vi "NI-DAQmxMulti.vi"() -> (0 "error out":errorcluster)   [LabVIEW 2022 SP3]
uses:
  Device ID port info.ctl
  Sub_vis/Upload Data.ctl
  <vilib>/DAQmx/read.llb/DAQmx Read (Analog 2D DBL NChan NSamp).vi
  Globals/Meas_global.vi
  <vilib>/DAQmx/miscellaneous.llb/DAQmx Fill In Error Info.vi
  <resource>/objmgr/daqmx.rc
panel:
  out "errorLog":T1(array[cluster])
  out "FsArray":dbl[](array[numeric]) format="%_12g"
  out "combinedTasks":string[](array[string])
  out "Device port info":T2[](array[typedef])
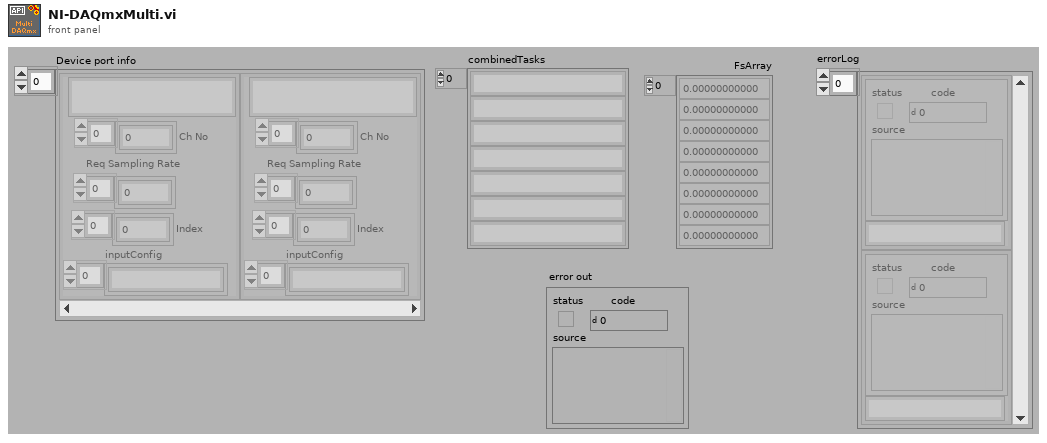
[diagram p1: front panel]
types:
  T1 = cluster{"error out":errorcluster, "String":string}[]
  T2 = typedef "Device ID port info.ctl" = cluster{"Ch No":i16[], "Req Sampling Rate":dbl[], "Port":string, "Index":i32[], "inputConfig":string[]}
  T3 = typedef "Analysis_info_cluster.ctl" = cluster{"Colour":u32, "Inst type":T4, "Inst name":string, "Symbol":string, "Code name":string, "Extra Info":string, "Inst Array":T5, "U":dbl, "u^2":dbl, "u^3":dbl, "u^4":dbl, "Skew_u":dbl, "Kurt_u":dbl, "Sd Error in Mean":dbl, "% u'/U":dbl, "X":dbl, "Y":dbl, "Z":dbl, "Timescale integral Estimate":dbl, "Sd Error in Variance":dbl, "Calib File":path, "Calib Constants":dbl[], "Output Position":bool, "Stats":enum16{"None", "Basic", "Full"}, "Av Sampling Rate":dbl, "Av No of Samples":dbl, "Total Meas Time (s)":dbl, "OrigChName":string, "Max value":dbl, "Min value":dbl, "Req Sample Rate Hz":dbl, "Sync Delay Time (s)":dbl, "Ch No":i16, "Device":string, "Use Latest Calib":bool, "Port":string, "Metadata Ch Names":string[], "Metadata Ch Values":string[], "Label":string, "chState":T6, "Point Drift":dbl, "inputConfig":string}
  T4 = typedef "Inst_type.ctl" = enum16{"Raw voltage", "Raw with zero offsetting", "Propeller anemometer", "Pressure Transducer", "Pitot-static tube", "Hot wire", "Cross wire 1", "Cross wire 2", "Generic Linear", "Generic Polynomial", "Generic BackPoly", "Fast FID", "Thermocouple", "Cold wire", "Pulsed Wire", "LDA Vel", "LDA Tran time", "LDA Arr time", "Microphone"}
  T5 = typedef "Instrument_Array.ctl" = enum16{"PWA", "LDA", "Analogue"}
  T6 = typedef "channelState.ctl" = enum32{"No Selection", "Solo", "Mute"}
  T7 = typedef "Upload Data.ctl" = enum16{"Voltage Array", "Time Trace Cluster"}
  T8 = typedef "Rendezvous RefNum" = refnum<k1>
  T9 = typedef "Setup.ctl" = enum16{"Run Program", "Show Setup", "Save Current Setup", "Setup Front Panel"}
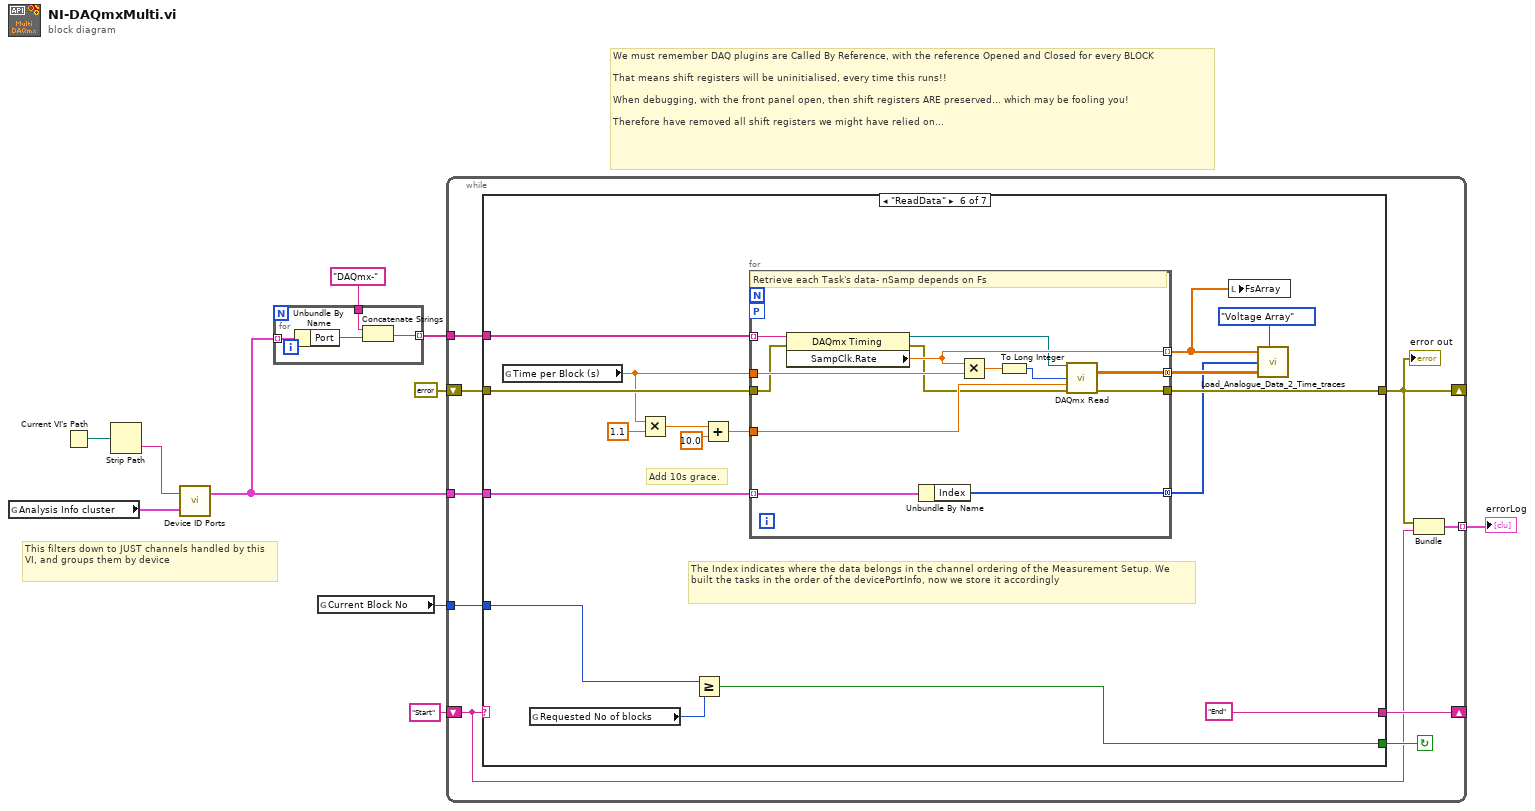
[diagram p0: block diagram]
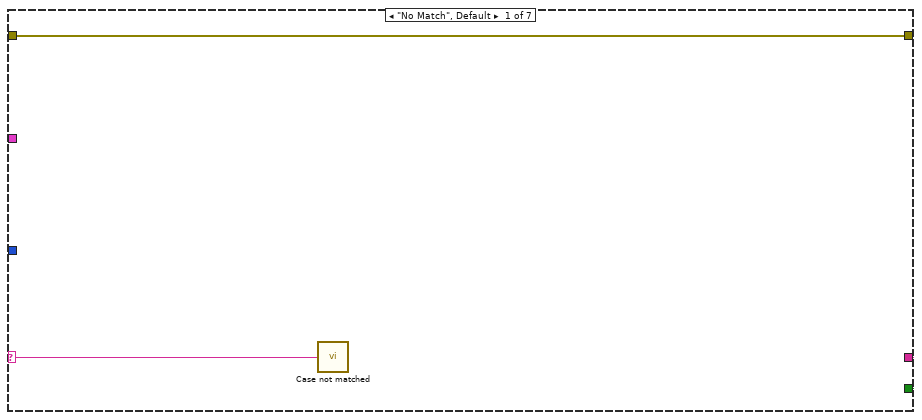
[diagram p2: hidden frame]
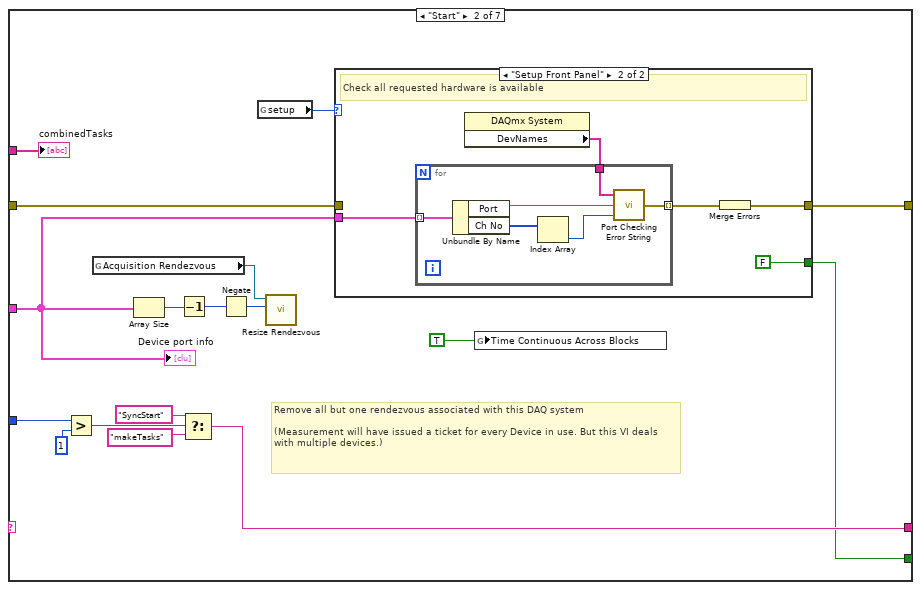
[diagram p3: hidden frame]
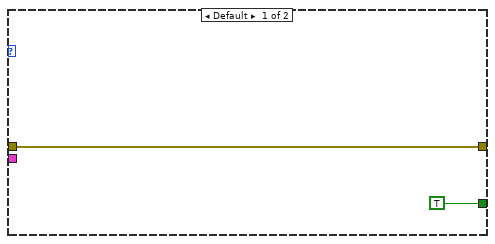
[diagram p4: hidden frame]
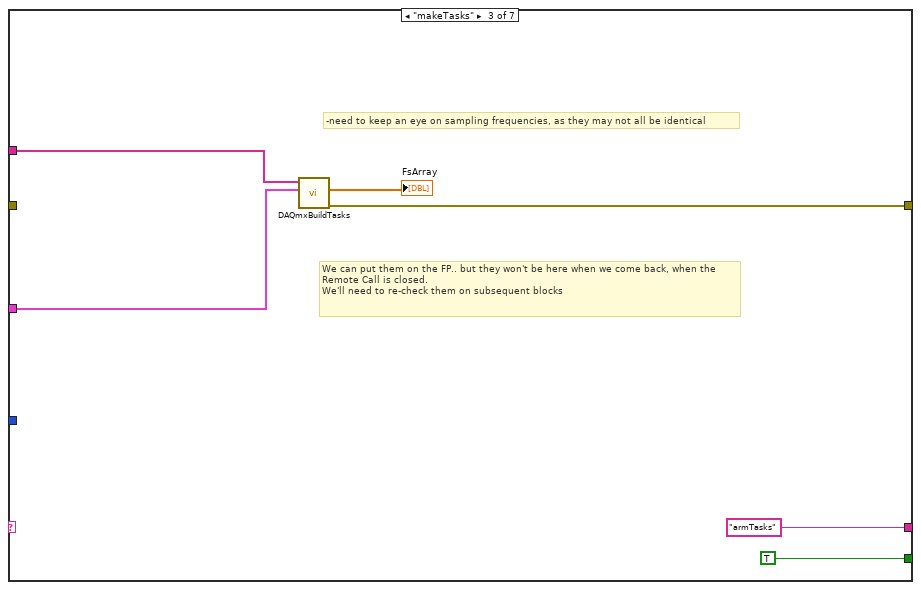
[diagram p5: hidden frame]
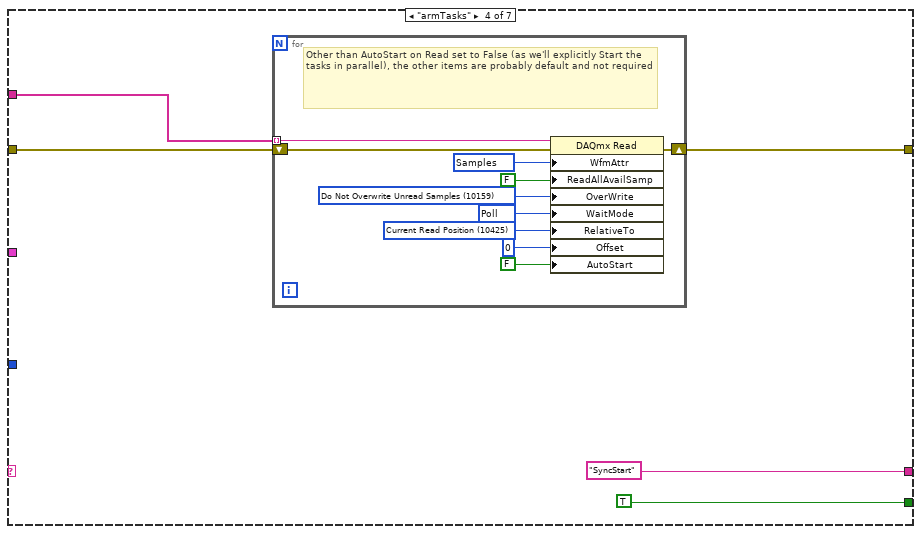
[diagram p6: hidden frame]
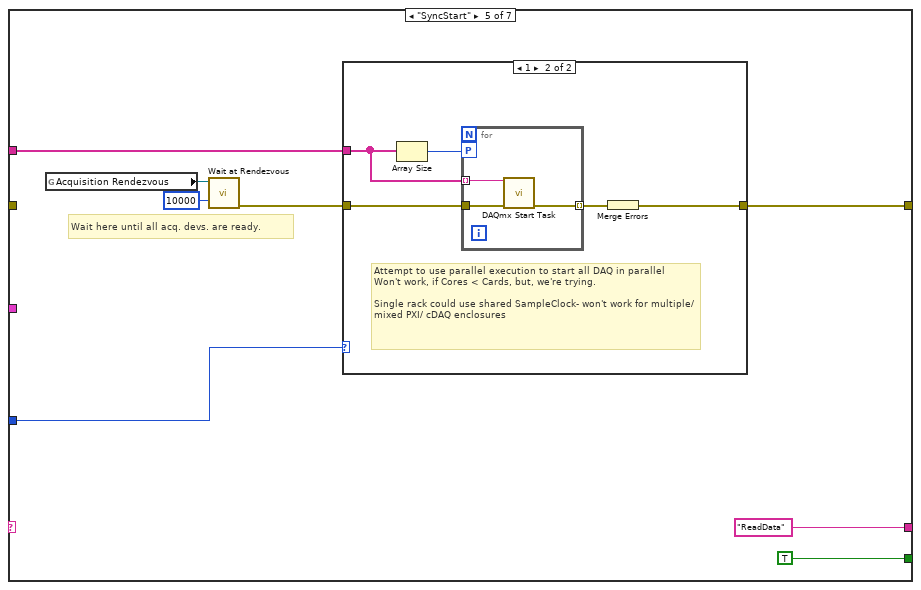
[diagram p7: hidden frame]
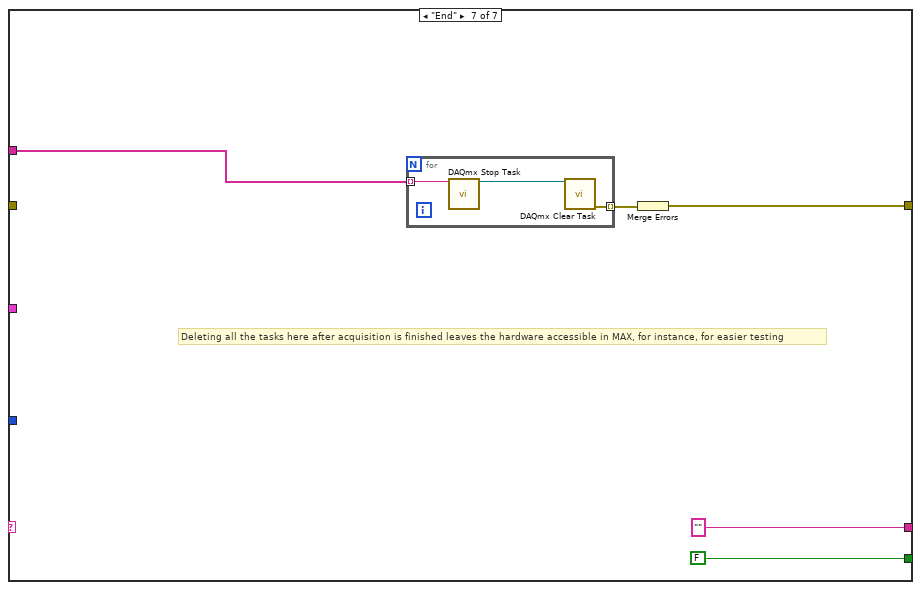
[diagram p9: hidden frame]
diagram:
  # "We must remember DAQ plugins are Called By Reference, with the reference Opened and Closed for every BLOCK\n\nThat means shift registers will be uninitialised, every time this runs!!\n\nWhen debugging, with the front panel open, then shift registers ARE preserved... which may be fooling you!\n\nTherefore have removed all shift registers we might have relied on..."
  # "This filters down to JUST channels handled by this VI, and groups them by device"
  n1 = global read "Meas_global.vi" "Analysis Info cluster"() -> (w6:T3[])
  n2 = Current VI's Path() -> (path=w9:path)
  n3 = Strip Path(path=w9) -> (name=w8:string)  [unwired: 1 out]
  n4 = call "Device ID Ports.vi"("Analysis Info cluster"=w6, "DAQdeviceType"=w8) -> ("Device port info"=w4:T2[])  [unwired: 1 out]
  n5 = for {
    tunnel: [w13] -> w3 mode=indexing
    tunnel: w4 -> [w12] mode=indexing
    tunnel: "DAQmx-" ("new task name") -> [w11]
    n6 = Unbundle By Name(w12) -> ("Port"=w14:string)
    n7 = Concatenate Strings(w11, w14) -> (w13:string)
  }
  n8 = global read "Meas_global.vi" "Current Block No"() -> (w7:i32)
  n9 = while {
    shift-left: "Start" -> [w16]
    shift-right: [w21] -> _
    shift-right: [w17] -> _
    shift-left: errorcluster {"status"=FALSE, "code"=0, "source"=""} ("error out") -> [w23]
    tunnel: w7 -> [w22]
    tunnel: w4 -> [w19]
    tunnel: w3 -> [w18]
    tunnel: [w15] -> w2 mode=indexing
    stop <- w20 continue-if-true
    n10 = case shown="\"ReadData\"" w16 {
      selector: w16 -> [w24 _ _ _ _ _ _]
      tunnel: [FALSE w40 TRUE TRUE TRUE w108 FALSE] -> w20
      tunnel: ["Initialise" w44 "armTasks" "SyncStart" "ReadData" ("f") "End" "" ("f")] -> w21
      tunnel: w23 -> [w25 w33 _ w64 _ w112 _]
      tunnel: w22 -> [_ w43 _ _ w79 w105 _]
      tunnel: w18 -> [_ w30 w60 w65 w82 w109 w128]
      tunnel: w19 -> [_ w29 w61 _ _ w107 _]
      tunnel: [w25 w41 w59 w66 w83 w110 w126] -> w17
      frame "No Match", Default {
        n11 = call "Case not matched.vi"("Case Name not Matched"=w24) -> ()
      }
      frame "Start" {
        # "Remove all but one rendezvous associated with this DAQ system\n\n(Measurement will have issued a ticket for every Device in use. But this VI deals with multiple devices.)"
        n12 = Greater?(x=w43, y=1) -> (0:w38:bool)
        n13 = global read "Meas_global.vi" "Acquisition Rendezvous"() -> (w34:T8)
        n14 = Array Size(array=w29) -> (size(s)=w37:i32)
        n15 = Decrement(x=w37) -> (x-1=w36:i32)
        n16 = Select(t="SyncStart" ("f"), s=w38, f="makeTasks") -> (s? t:f=w44:string)
        n17 = Negate(x=w36) -> (-x=w35:i32)
        n18 = global read "Meas_global.vi" "setup"() -> (w42:T9)
        n19 = call <vilib>:"Resize Rendezvous.vi"("size change (0)"=w35, "rendezvous"=w34) -> ()  [unwired: 3 in, 3 out]
        n20 = case shown="\"Setup Front Panel\"" w42 {
          tunnel: [w45 w47] -> w41
          tunnel: [TRUE FALSE] -> w40
          tunnel: w29 -> [_ w48]
          tunnel: w33 -> [w45 _]
          frame Default {
          }
          frame "Setup Front Panel" {
            # "Check all requested hardware is available"
            n21 = property class="DAQmx System"() -> ("DevNames"=w51:tag[])  [unwired: 2 in, 2 out]
            n22 = for {
              tunnel: w51 -> [w57]
              tunnel: [w56] -> w50 mode=indexing
              tunnel: w48 -> [w55] mode=indexing
              n23 = Unbundle By Name(w55) -> ("Port"=w54:string, "Ch No"=w53:i16[])
              n24 = Index Array(array=w53) -> (element=w52:i16)  [unwired: 1 in]
              n25 = call "Port Checking Error String.vi"("Ch Index"=w52, "Port"=w54, "Available Ports"=w57) -> ("error out"=w56:errorcluster)  [unwired: 1 in]
            }
            n26 = Merge Errors(w50) -> (w47:errorcluster)
          }
        }
        n27 = global write "Meas_global.vi" "Time Continuous Across Blocks"(TRUE ("Time Continuous across Blocks")) -> ()
        "combinedTasks" <- w30
        "Device port info" <- w29
      }
      frame "makeTasks" {
        # "We can put them on the FP.. but they won't be here when we come back, when the Remote Call is closed.\nWe'll need to re-check them on subsequent blocks"
        # "-need to keep an eye on sampling frequencies, as they may not all be identical"
        n28 = call "DAQmxBuildTasks.vi"("Device port info"=w61, "taskNamesIn"=w60) -> ("error out"=w59:errorcluster, "FsOut"=→"FsArray":dbl[])  [unwired: 8 in]
      }
      frame "armTasks" {
        n29 = for {
          tunnel: w65 -> [w70] mode=indexing
          shift-right: [w71] -> w66
          shift-left: w64 -> [w69]
          w74 = 10425 items=["First Sample"=10424, "Current Read Position"=10425, "Reference Trigger"=10426, "First Pretrigger Sample"=10427, "Most Recent Sample"=10428] ("RelativeTo")
          w75 = 12524 items=["Wait For Interrupt"=12523, "Poll"=12524, "Yield"=12525, "Sleep"=12547] ("WaitMode")
          w76 = 10159 items=["Overwrite Unread Samples"=10252, "Do Not Overwrite Unread Samples"=10159] ("OverWrite")
          w78 = 10287 items=["Samples"=10287, "Samples and Timing"=10140, "Samples, Timing, and Attributes"=10141] ("WfmAttr")
          # "Other than AutoStart on Read set to False (as we'll explicitly Start the tasks in parallel), the other items are probably default and not required"
          n30 = property class="DAQmx Read"(reference=w70, error in=w69, "WfmAttr"=w78, "ReadAllAvailSamp"=FALSE, "OverWrite"=w76, "WaitMode"=w75, "RelativeTo"=w74, "Offset"=0, "AutoStart"=FALSE) -> (error out=w71:errorcluster)  [unwired: 1 out]
        }
      }
      frame "SyncStart" {
        # "Wait here until all acq. devs. are ready."
        n31 = global read "Meas_global.vi" "Acquisition Rendezvous"() -> (w86:T8)
        n32 = call <vilib>:"Wait at Rendezvous.vi"("ms timeout (-1)"=10000, "rendezvous"=w86) -> ("error out"=w84:errorcluster)  [unwired: 3 in, 2 out]
        n33 = case shown="1" w79 {
          tunnel: w84 -> [w87 w91]
          tunnel: [w87 w90] -> w83
          tunnel: w82 -> [_ w88]
          frame 2, Default {
          }
          frame 1 {
            # "Attempt to use parallel execution to start all DAQ in parallel\nWon't work, if Cores < Cards, but, we're trying.\n\nSingle rack could use shared SampleClock- won't work for multiple/ mixed PXI/ cDAQ enclosures"
            n34 = Array Size(array=w88) -> (size(s)=w89:i32)
            n35 = for {
              tunnel: w88 -> [w95] mode=indexing
              workers-P: w89 -> [_]
              tunnel: [w94] -> w92 mode=indexing
              tunnel: w91 -> [w93]
              n36 = call <vilib>:"DAQmx Start Task.vi"("task/channels in"=w95, "error in"=w93) -> ("error out"=w94:errorcluster)  [unwired: 12 in, 1 out]
            }
            n37 = Merge Errors(w92) -> (w90:errorcluster)
          }
        }
      }
      frame "ReadData" {
        # "Add 10s grace."
        # "The Index indicates where the data belongs in the channel ordering of the Measurement Setup. We built the tasks in the order of the devicePortInfo, now we store it accordingly"
        n38 = global read "Meas_global.vi" "Time per Block (s)"() -> (w99:dbl)
        n39 = global read "Meas_global.vi" "Requested No of blocks"() -> (w106:i32)
        n40 = Multiply(x=w99, y=1.1) -> (x*y=w98:dbl)
        n41 = Greater Or Equal?(x=w105, y=w106) -> (x >= y?=w108:bool)
        n42 = Add(x=w98, y=10.0) -> (x+y=w102:dbl)
        n43 = for {
          tunnel: w112 -> [w113]
          tunnel: w102 -> [w124]
          tunnel: [w125] -> w110
          tunnel: w109 -> [w115] mode=indexing
          workers-P: _ -> [_]
          tunnel: [w123] -> w101 mode=concatenating
          tunnel: w107 -> [w122] mode=indexing
          tunnel: [w121] -> w100 mode=concatenating
          tunnel: w99 -> [w119]
          tunnel: [w117] -> w96 mode=indexing
          # "Retrieve each Task's data- nSamp depends on Fs"
          n44 = property class="DAQmx Timing"(reference=w115, error in=w113) -> (reference out=w116:refnum<k21>, error out=w114:errorcluster, "SampClk.Rate"=w117:dbl)
          n45 = Unbundle By Name(w122) -> ("Index"=w121:i32[])
          n46 = Multiply(x=w117, y=w119) -> (x*y=w120:dbl)
          n47 = To Long Integer(number=w120) -> (32bit integer=w118:i32)
          n48 = call-poly <vilib>:"DAQmx Read.vi"("task/channels in"=w116, "number of samples per channel"=w118, "timeout"=w124, "error in"=w114) -> ("data"=w123:dbl[][], "error out"=w125:errorcluster)  [unwired: 10 out]
        }
        n49 = local write "FsArray"(w96) -> ()
        n50 = call "Load_Analogue_Data_2_Time_traces.vi"("Sampling Rate (Hz)"=w96, "Mode"=Upload_Data."Voltage Array", "Index"=w100, "Voltage Array"=w101) -> ()  [unwired: 3 in]
      }
      frame "End" {
        # "Deleting all the tasks here after acquisition is finished leaves the hardware accessible in MAX, for instance, for easier testing"
        n51 = for {
          tunnel: w128 -> [w133] mode=indexing
          tunnel: [w131] -> w127 mode=indexing
          n52 = call <vilib>:"DAQmx Stop Task.vi"("task/channels in"=w133) -> ("task out"=w132:refnum<k21>)  [unwired: 13 in, 1 out]
          n53 = call <vilib>:"DAQmx Clear Task.vi"("task in"=w132) -> ("error out"=w131:errorcluster)  [unwired: 1 in, 13 out]
        }
        n54 = Merge Errors(w127) -> (w126:errorcluster)
      }
    }
    "error out" <- w17
    n55 = Bundle("error IO"=w17, w16) -> (w15:cluster{"error IO":errorcluster, string})  [unwired: 1 in]
  }
  "errorLog" <- w2
